vi "SensorsOperations.vi"(8 "ErrorIn":errorcluster, 9 "Operation":T1, 10 "RawAccelerationData In":dbl[][](array[numeric]), 11 "frame length ms":i64=50) -> (0 "ErrorOut":errorcluster, 1 "Tachometer Data":dbl[](array[numeric]), 2 "Normalized Acceleration Data":dbl[][](array[numeric]), 3 "RawAccelerationData Out":dbl[][](array[numeric]))   [LabVIEW 2019]
uses:
  Operation.ctl
  <vilib>/myRIO/Instrument Drivers/Onboard IO/AI/typedefs/AI Reference.ctl
  <vilib>/myRIO/Common/Instrument Driver Framework/Utilities/typedefs/myRIO Generic Hardware Reference.ctl
  <vilib>/myRIO/Common/Instrument Driver Framework/Utilities/typedefs/Hardware Version Enum.ctl
  <vilib>/myRIO/Common/Instrument Driver Framework/Utilities/typedefs/myRIO v1.0 Reference.ctl
  <vilib>/myRIO/Common/Instrument Driver Framework/Utilities/typedefs/Generic FPGA Reference.ctl
  <vilib>/myRIO/Common/Instrument Driver Framework/myRIO v1.0/AI/typedefs/AI Channels List.ctl
  <vilib>/myRIO/Common/Instrument Driver Framework/myRIO v1.0/AI/typedefs/AI Channels Enum.ctl
  <vilib>/myRIO/Common/Instrument Driver Framework/Utilities/typedefs/Analog Scaling Constants List.ctl
  <vilib>/myRIO/Common/Instrument Driver Framework/Utilities/typedefs/Analog Scaling Constants.ctl
  <vilib>/userdefined/High Color/nirio_resource_hc.ctl
  <vilib>/Platform/TimedLoop/XDataNode/timing_clust.ctl
  <vilib>/Platform/TimedLoop/XDataNode/nitl_modes.ctl
  <vilib>/Platform/TimedLoop/XDataNode/wakeup.ctl
  <vilib>/myRIO/Instrument Drivers/Onboard IO/I2C/typedefs/I2C Reference.ctl
  <vilib>/myRIO/Common/Instrument Driver Framework/myRIO v1.0/I2C/typedefs/I2C Channels Enum.ctl
  <vilib>/myRIO/Instrument Drivers/Onboard IO/I2C/typedefs/I2C Configuration.ctl
  <vilib>/myRIO/Instrument Drivers/Onboard IO/I2C/typedefs/I2C Transfer Rate.ctl
  <vilib>/myRIO/Common/Instrument Driver Framework/myRIO v1.0/AI/vis/myRIO v1.1 Open Throughput AI.vi
  <vilib>/myRIO/Common/Instrument Driver Framework/Utilities/vis/Validate Channels.vi
  <vilib>/myRIO/Common/Instrument Driver Framework/myRIO v1.0/AI/vis/myRIO v1.0 Reserve AI.vi
  <vilib>/myRIO/Common/Instrument Driver Framework/myRIO v1.0/I2C/vis/myRIO v1.0 Close I2C.vi
  <vilib>/myRIO/Common/Instrument Driver Framework/myRIO v1.0/AI/vis/myRIO v1.0 Close AI.vi
  <vilib>/myRIO/Common/Instrument Driver Framework/myRIO v1.0/AI/vis/myRIO v1.0 Build MUX Configuration AI.vi
  <vilib>/myRIO/Common/Instrument Driver Framework/myRIO v1.0/Resource Manager/vis/myRIO v1.0 Reserve Channel List.vi
  <vilib>/myRIO/Common/Instrument Driver Framework/myRIO v1.0/I2C/vis/myRIO v1.0 Unreserve I2C.vi
  <vilib>/myRIO/Common/Instrument Driver Framework/myRIO v1.0/AI/vis/myRIO v1.0 Unreserve AI.vi
  <vilib>/myRIO/Common/Instrument Driver Framework/myRIO v1.0/Resource Manager/vis/myRIO v1.0 Reserve Channel.vi
  <vilib>/myRIO/Common/Instrument Driver Framework/myRIO v1.0/Resource Manager/vis/myRIO v1.0 Unreserve Channel.vi
  <vilib>/myRIO/Common/Instrument Driver Framework/myRIO v1.0/I2C/vis/myRIO v1.0 Build MUX Configuration I2C.vi
  <vilib>/myRIO/Common/Instrument Driver Framework/myRIO v1.0/Resource Manager/vis/myRIO v1.0 Unreserve Channel List.vi
  <vilib>/myRIO/Common/Instrument Driver Framework/myRIO v1.0/Resource Manager/vis/myRIO v1.0 Build Mutex Name.vi
  <vilib>/myRIO/Common/Instrument Driver Framework/myRIO v1.0/Resource Manager/vis/myRIO v1.0 Create Configuration List.vi
  <vilib>/Utility/VariantDataType/GetNumericInfo.vi
  <vilib>/Utility/error.llb/Error Cluster From Error Code.vi
  <vilib>/myRIO/Common/Instrument Driver Framework/myRIO v1.0/myRIO v1.1 Open Throughput.vi
  <vilib>/myRIO/Common/Instrument Driver Framework/myRIO v1.0/AI/vis/myRIO v1.0 Get Scaling Constants AI.vi
  <vilib>/myRIO/Common/Instrument Driver Framework/Utilities/vis/IO Manager.vi
  <vilib>/myRIO/Common/Instrument Driver Framework/Utilities/vis/Configuration Manager.vi
  <vilib>/myRIO/Common/Instrument Driver Framework/myRIO v1.0/myRIO v1.0 Close.vi
  <vilib>/myRIO/Common/Instrument Driver Framework/myRIO v1.0/AI/vis/myRIO v1.0 Read AI.vi
  <vilib>/myRIO/Common/Instrument Driver Framework/myRIO v1.0/I2C/vis/myRIO v1.0 Shutdown I2C.vi
  <vilib>/myRIO/Common/Instrument Driver Framework/myRIO v1.0/Resource Manager/vis/myRIO v1.0 Configure IO.vi
  <vilib>/myRIO/Instrument Drivers/Onboard IO/AI/vis/myRIO AI Open.xnode
  <vilib>/platform/TimedLoop/XDataNode/XDataNode.xnode
  <vilib>/myRIO/Instrument Drivers/Onboard IO/I2C/typedefs/I2C User Configuration.ctl
  <vilib>/myRIO/Instrument Drivers/Onboard IO/I2C/I2C.lvlib
  <vilib>/myRIO/Instrument Drivers/Onboard IO/I2C/vis/myRIO I2C Open.xnode
  <vilib>/myRIO/Instrument Drivers/Onboard IO/AI/AI.lvlib
  <vilib>/Platform/TimedLoop/XDataNode/XDNodeRunTimeDep.lvlib
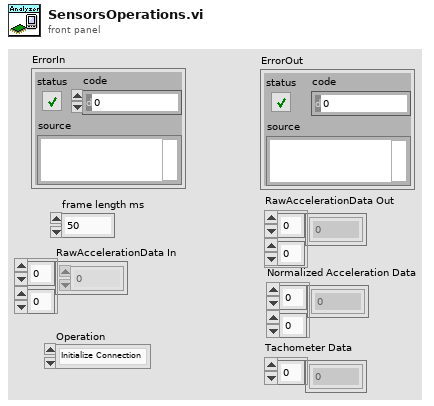
[diagram p1: front panel]
types:
  T1 = typedef "Operation.ctl" = enum16{"Initialize Connection", "Read Data", "Close Connection", "Calculate Data To g"}
  T2 = typedef "AnalyzerSettings.ctl" = cluster{"Create NS Timeout Code":i32, "Destroy NS Timeout Code":i32, "All threads":T3[], "AnalysisSettings":T4}
  T3 = typedef "AThreads.ctl" = enum16{"UI", "analyzeAccelerationData", "aquireAccelerationData", "communicateWebServices", "TDMSmanager", "aquireTachoSignal"}
  T4 = typedef "AnalysisSettings.ctl" = cluster{"Fault Thresholds":T5, "Analysis series name":string, "Save data analysis?":bool, "Band size":i32, "OrderAnalysis?":bool, "Accelerometer":T7, "fs [Hz]":dbl}
  T5 = typedef "Thresholds.ctl" = cluster{"Parameters labels":T6[], "Parameters thresholds":dbl[], "Freqs and thresholds":dbl[][], "Orders and thresholds":dbl[][]}
  T6 = typedef "FaultParameter.ctl" = enum16{"Kurtosis", "RMS", "Crest factor"}
  T7 = typedef "Accelerometer.ctl" = enum16{"None", "MPU6050", "MMA7351"}
  T8 = typedef "nirio_resource_hc.ctl" = tag
  T9 = typedef "Hardware Version Enum.ctl" = enum16{"Unknown", "myRIO-1900", "myRIO-1950", "roboRIO", "NI ELVIS RIO CM", "ELVIS III"}
  T10 = typedef "XDNodeRunTimeDep.lvlib/timing_clust.ctl" = cluster{"Expected End [f-1]":u64, "Actual End [f-1]":u64, "Finished Late? [f-1]":bool, "Expected End [i-1]":u64, "Actual End [i-1]":u64, "Finished Late? [i-1]":bool, "Expected Start [i]":u64, "Actual Start [i]":u64, "Expected Start [f]":u64, "Actual Start [f]":u64, "Source Name":string, "Structure Name":string, "Period":i64, "Deadline":i64, "Offset":i64, "Start":i64, "Priority":i32, "Timeout":i32, "Mode":T11, "Wakeup Reason":T12, "Error":errorcluster, "Source Type":string, "Secondary Source Type":string, "Global End Time":u64, "Global Start Time":u64, "Frame Duration":u64, "Iteration Duration":u64, "Assigned CPU":i32, "I/O Scan Engine Mode":u32}
  T11 = typedef "XDNodeRunTimeDep.lvlib/nitl_modes.ctl" = enum32{"No Change", "Process missed periods, maintain original phase", "Discard missed periods, maintain original phase", "Process missed periods, ignore original phase", "Discard missed periods, ignore original phase"}
  T12 = typedef "XDNodeRunTimeDep.lvlib/wakeup.ctl" = enum32{"Normal", "Aborted", "Asynchronous wakeup", "Timing source error", "Timed loop error", "Timeout"}
  T13 = typedef "I2C.lvlib/I2C Reference.ctl" = cluster{"myRIO Reference":T14, "I2C Channels Enum":T17, "I2C Configuration":T18}
  T14 = typedef "myRIO Generic Hardware Reference.ctl" = cluster{"myRIO Model":T9, "myRIO Hardware Reference":T15}
  T15 = typedef "myRIO v1.0 Reference.ctl" = cluster{"Generic FPGA Reference":T16, "Allow multiple opens":bool}
  T16 = typedef "Generic FPGA Reference.ctl" = refnum<k20>
  T17 = typedef "I2C Channels Enum.ctl" = enum16{"Not Connected", "A/I2C", "B/I2C", "I2C/I2C"}
  T18 = typedef "I2C.lvlib/I2C Configuration.ctl" = cluster{"I2C Transfer Rate":T19}
  T19 = typedef "I2C.lvlib/I2C Transfer Rate.ctl" = enum16{"Standard mode (100 kbps)", "Fast mode (400 kbps)"}
  T20 = typedef "AI.lvlib/AI Reference.ctl" = cluster{"myRIO Reference":T14, "AI Channels List":T21, "AI Scaling Constants List":T23}
  T21 = typedef "AI Channels List.ctl" = T22[]
  T22 = typedef "AI Channels Enum.ctl" = enum16{"Not Connected", "AudioIn/Left", "AudioIn/Right", "C/AI0", "C/AI1", "A/AI0", "A/AI1", "A/AI2", "A/AI3", "A/AI4", "A/AI5", "A/AI6", "A/AI7", "B/AI0", "B/AI1", "B/AI2", "B/AI3", "B/AI4", "B/AI5", "B/AI6", "B/AI7", "AI/AI0", "AI/AI1", "AI/AI2", "AI/AI3", "A/AI0 (DIFF)", "A/AI1 (DIFF)", "A/AI2 (DIFF)", "A/AI3 (DIFF)", "B/AI0 (DIFF)", "B/AI1 (DIFF)", "B/AI2 (DIFF)", "B/AI3 (DIFF)"}
  T23 = typedef "Analog Scaling Constants List.ctl" = T24[]
  T24 = typedef "Analog Scaling Constants.ctl" = cluster{"LSB Weight (Volts)":dbl, "Offset (Volts)":dbl, "Signed?":bool}
  T25 = typedef "I2C.lvlib/I2C User Configuration.ctl" = cluster{"I2C Transfer Rate":T19}
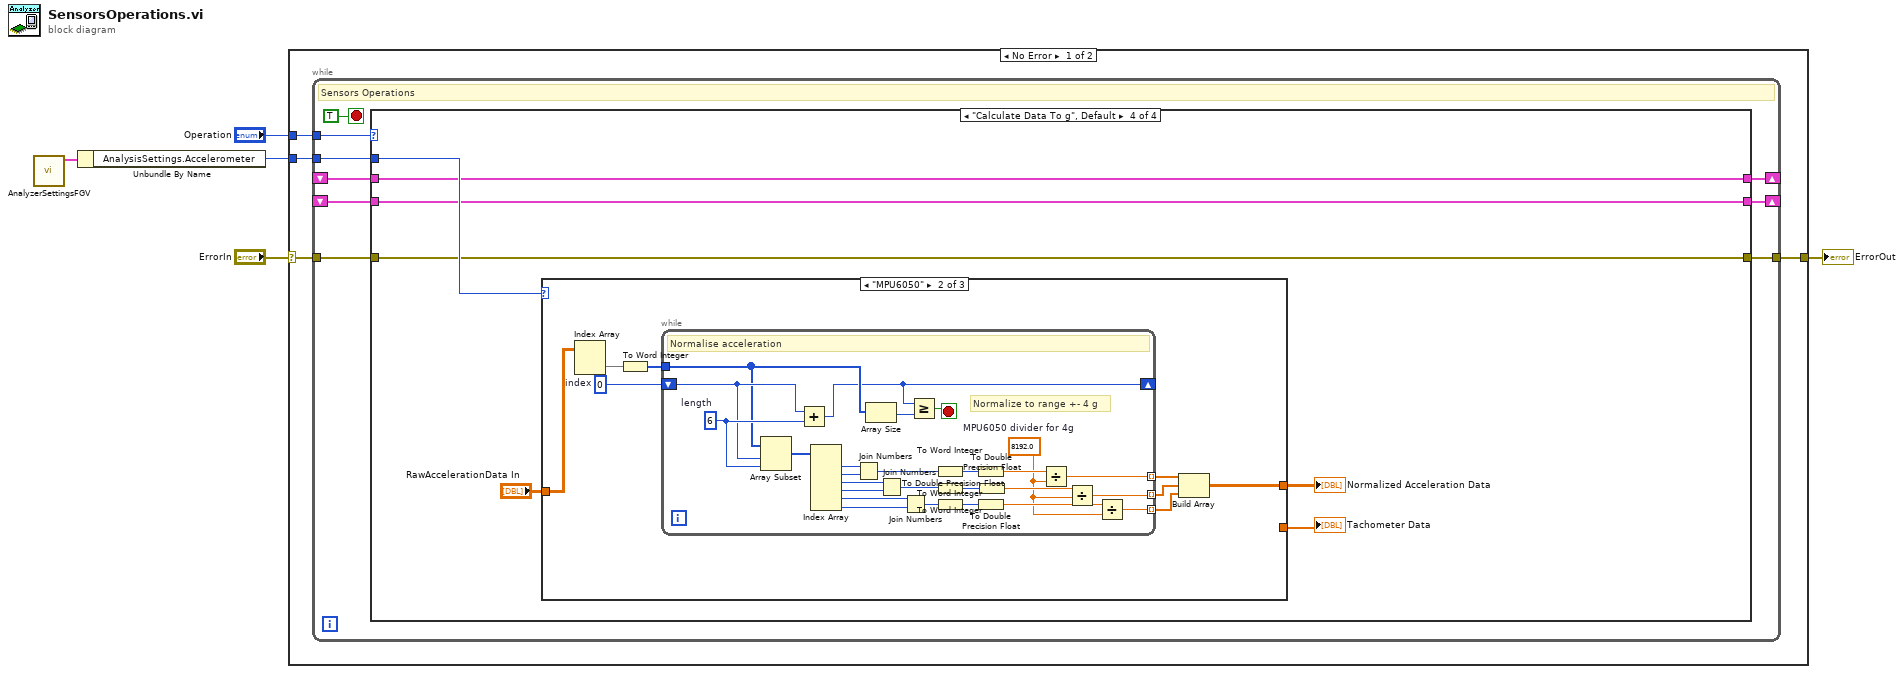
[diagram p0: block diagram]
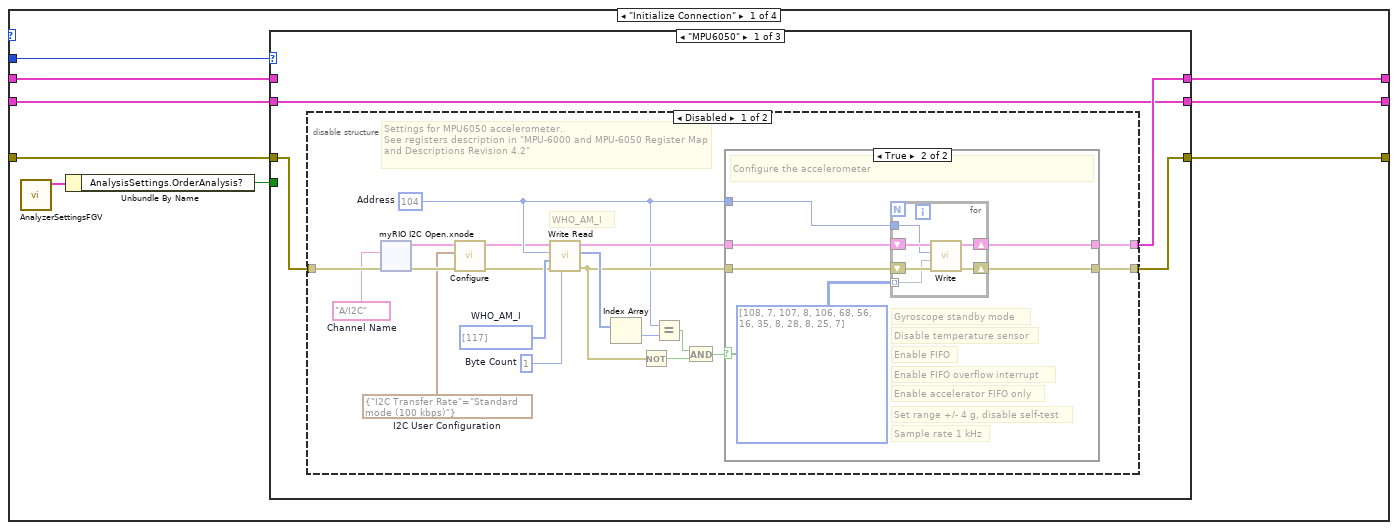
[diagram p2: hidden frame]
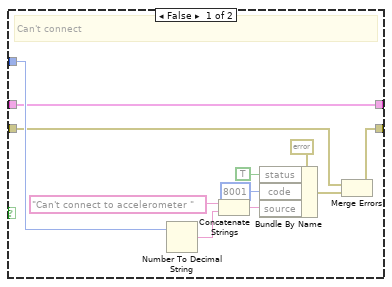
[diagram p3: hidden frame]
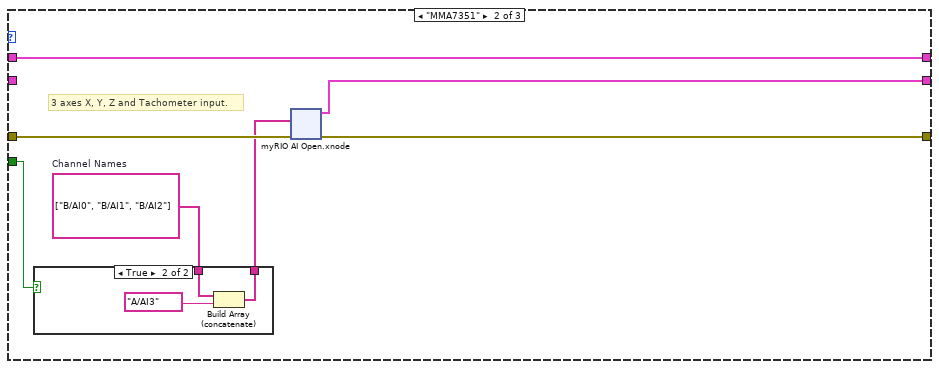
[diagram p5: hidden frame]
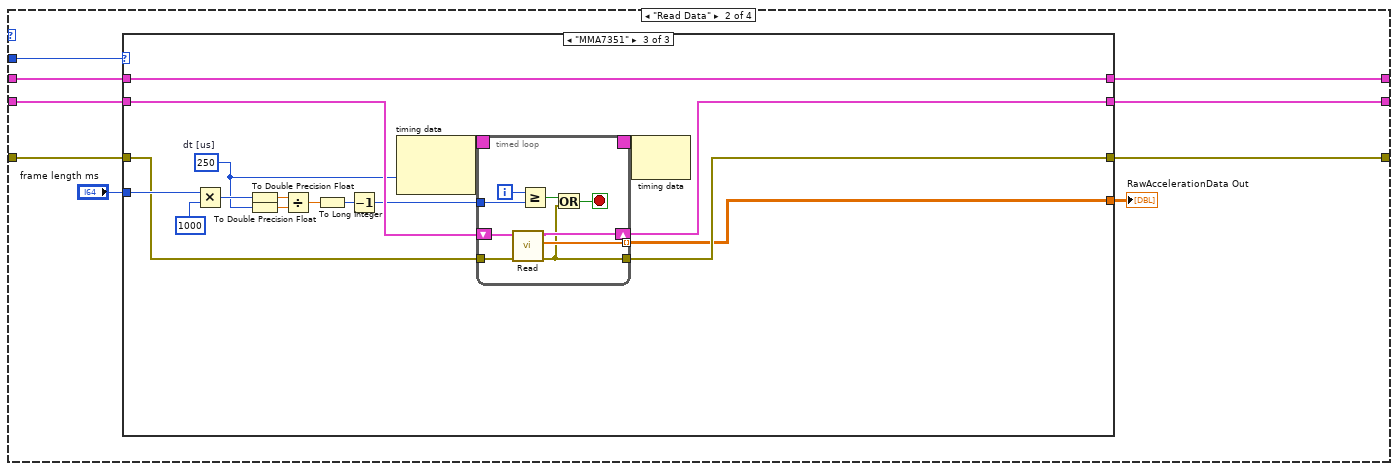
[diagram p8: hidden frame]
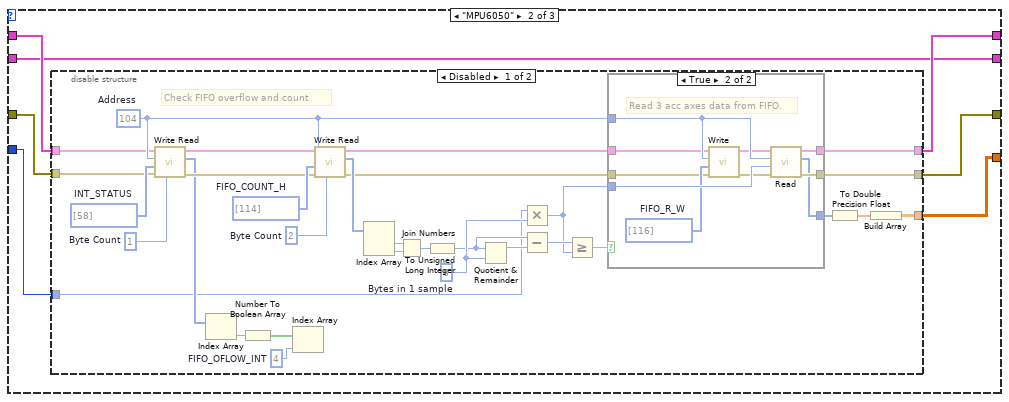
[diagram p10: hidden frame]
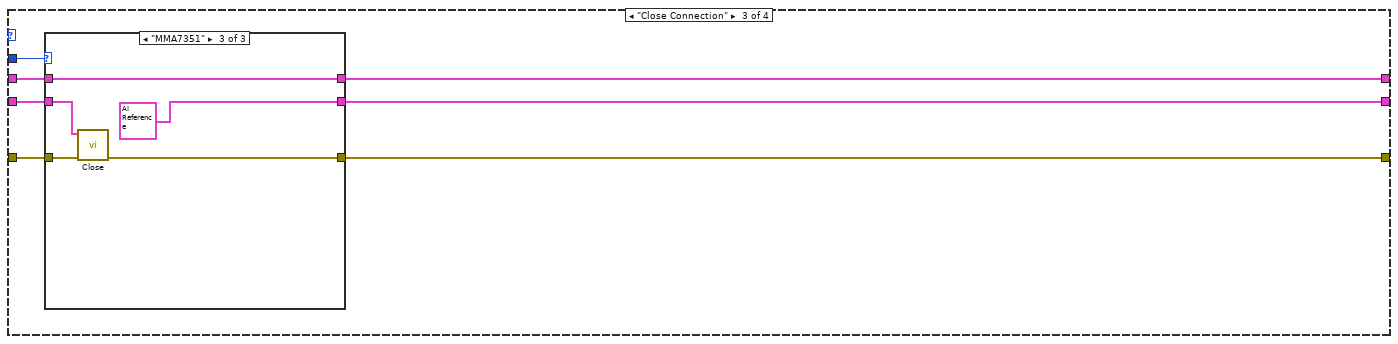
[diagram p13: hidden frame]
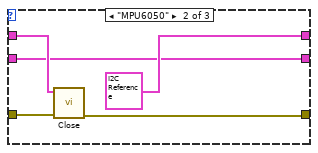
[diagram p15: hidden frame]
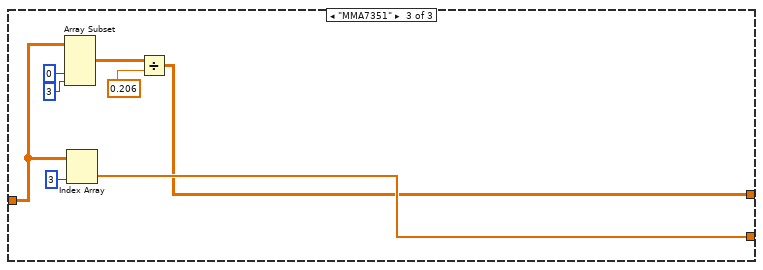
[diagram p17: hidden frame]
diagram:
  n1 = call "AnalyzerSettingsFGV.vi"() -> ("GlobalSettingsOut"=w3:T2)  [unwired: 11 in]
  n2 = Unbundle By Name(w3) -> ("AnalysisSettings.Accelerometer"=w2:T7)
  n3 = case shown="No Error" "ErrorIn" {
    selector: "ErrorIn" -> [w6 w272]
    tunnel: "Operation" -> [w9 _]
    tunnel: [w8 w272] -> w4
    tunnel: w2 -> [w7 _]
    frame No Error {
      n4 = while {
        tunnel: w9 -> [w17]
        tunnel: w7 -> [w16]
        shift-right: [w12] -> _
        shift-left: _ -> [w13]
        shift-right: [w11] -> _
        shift-left: _ -> [w10]
        tunnel: w6 -> [w15]
        tunnel: [w14] -> w8
        stop <- TRUE stop-if-true
        # "Sensors Operations"
        n5 = case shown="\"Calculate Data To g\", Default" w17 {
          tunnel: w16 -> [w27 w115 w208 w228]
          tunnel: w15 -> [w26 w113 w204 w224]
          tunnel: [w25 w114 w205 w224] -> w14
          tunnel: w13 -> [w24 w112 w207 w222]
          tunnel: [w23 w109 w202 w222] -> w12
          tunnel: [w22 w108 w203 w223] -> w11
          tunnel: w10 -> [w21 w111 w206 w223]
          frame "Initialize Connection" {
            n6 = call "AnalyzerSettingsFGV.vi"() -> ("GlobalSettingsOut"=w20:T2)  [unwired: 11 in]
            n7 = Unbundle By Name(w20) -> ("AnalysisSettings.OrderAnalysis?"=w19:bool)
            n8 = case shown="\"MPU6050\"" w27 {
              tunnel: w26 -> [w30 w81 w106]
              tunnel: [w29 w80 w106] -> w25
              tunnel: w24 -> [_ w75 w104]
              tunnel: [w31 w75 w104] -> w23
              tunnel: [w28 w79 w105] -> w22
              tunnel: w21 -> [w28 _ w105]
              tunnel: w19 -> [_ w78 _]
              frame "MPU6050" {
                n9 = disable-structure shown="Disabled" {
                  disable-tunnel: [w40 _] -> w31
                  disable-tunnel: w30 -> [w39 w74]
                  disable-tunnel: [w32 w74] -> w29
                  frame Disabled {
                    w33 = T25 {"I2C Transfer Rate"=enum."Standard mode (100 kbps)"}  # I2C User Configuration
                    w38 = tag "A/I2C"  # Channel Name
                    w42 = u8 104  # Address
                    w48 = u32 1  # Byte Count
                    w47 = u8[] [117]  # WHO_AM_I
                    # "Settings for MPU6050 accelerometer.\nSee registers description in \"MPU-6000 and MPU-6050 Register Map and Descriptions Revision 4.2\""
                    # "WHO_AM_I"
                    n10 = xnode "myRIO I2C Open.xnode"("error in (no error)"=w39, "Channel Name"=w38) -> ("error out"=w36:errorcluster, "I2C Ref Out"=w37:T13)  [unwired: 1 in]
                    n11 = call <vilib>:"Configure.vi"("error in (no error)"=w36, "I2C User Configuration"=w33, "I2C Ref In"=w37) -> ("error out"=w34:errorcluster, "I2C Ref Out"=w35:T13)  [unwired: 7 in]
                    n12 = call <vilib>:"Write Read.vi"("Byte Count"=w48, "error in (no error)"=w34, "Bytes to Write"=w47, "Slave Address (7-bit)"=w42, "I2C Ref In"=w35) -> ("error out"=w44:errorcluster, "Bytes Read"=w49:u8[], "I2C Ref Out"=w46:T13)  [unwired: 3 in]
                    n13 = Index Array(array=w49) -> (element=w50:u8)  [unwired: 1 in]
                    n14 = Not(x=w44) -> (.not. x?=w43:bool)
                    n15 = Equal?(x=w42, y=w50) -> (x = y?=w45:bool)
                    n16 = And(x=w45, y=w43) -> (x .and. y?=w41:bool)
                    n17 = case shown="True" w41 {
                      tunnel: w42 -> [w59 w64]
                      tunnel: w46 -> [w52 w67]
                      tunnel: w44 -> [w54 w66]
                      tunnel: [w51 w63] -> w32
                      tunnel: [w52 w62] -> w40
                      frame False {
                        # "Can't connect"
                        n18 = Number To Decimal String(number=w59) -> (decimal integer string=w56:string)  [unwired: 1 in]
                        n19 = Concatenate Strings("Can't connect to accelerometer " ("source"), w56) -> (w58:string)
                        n20 = Bundle By Name(cluster=errorcluster {"status"=FALSE, "code"=0, "source"=""} ("error constant"), "status"=TRUE, "code"=8001, "source"=w58) -> (w53:errorcluster)
                        n21 = Merge Errors(w54, w53) -> (w51:errorcluster)
                      }
                      frame True {
                        # "Sample rate 1 kHz"
                        # "Enable accelerator FIFO only"
                        # "Disable temperature sensor"
                        # "Gyroscope standby mode"
                        # "Set range +/- 4 g, disable self-test"
                        # "Enable FIFO"
                        # "Enable FIFO overflow interrupt"
                        # "Configure the accelerometer"
                        n22 = for {
                          shift-right: [w70] -> w63
                          shift-left: w66 -> [w73]
                          shift-right: [w71] -> w62
                          shift-left: w67 -> [w72]
                          tunnel: u8[][] [[108, 7], [107, 8], [106, 68], [56, 16], [35, 8], [28, 8], [25, 7]] ("Bytes to Write") -> [w69] mode=indexing
                          tunnel: w64 -> [w68]
                          n23 = call <vilib>:"Write.vi"("error in (no error)"=w73, "Bytes to Write"=w69, "Slave Address (7-bit)"=w68, "I2C Ref In"=w72) -> ("error out"=w70:errorcluster, "I2C Ref Out"=w71:T13)  [unwired: 6 in]
                        }
                      }
                    }
                  }
                  frame Enabled {
                  }
                }
              }
              frame "MMA7351" {
                w77 = tag[] ["B/AI0", "B/AI1", "B/AI2"]  # Channel Names
                # "3 axes X, Y, Z and Tachometer input."
                n24 = case shown="True" w78 {
                  tunnel: w77 -> [w82 w85]
                  tunnel: [w82 w83] -> w76
                  frame False {
                  }
                  frame True {
                    n25 = Build Array (concatenate)(w85, tag "A/AI3" ("myRIO AI Channel")) -> (w83:tag[])
                  }
                }
                n26 = xnode "myRIO AI Open.xnode"("error in (no error)"=w81, "Channel Names"=w76) -> ("error out"=w80:errorcluster, "AI Ref Out"=w79:T20)  [unwired: 1 in]
              }
              frame "None", Default {
              }
            }
          }
          frame "Read Data" {
            n27 = case shown="\"MMA7351\"" w115 {
              tunnel: [w118 w119 w173] -> w114
              tunnel: w113 -> [w118 w121 w175]
              tunnel: w112 -> [w116 w124 w170]
              tunnel: w111 -> [w117 w120 w177]
              tunnel: "frame length ms" -> [_ w125 w180]
              tunnel: [w116 w123 w170] -> w109
              tunnel: [_ w122 w172] -> w107
              tunnel: [w117 w120 w174] -> w108
              frame "None", Default {
              }
              frame "MPU6050" {
                n28 = disable-structure shown="Disabled" {
                  disable-tunnel: w121 -> [w133 w168]
                  disable-tunnel: w125 -> [w132 _]
                  disable-tunnel: [w131 w168] -> w119
                  disable-tunnel: w124 -> [w130 w169]
                  disable-tunnel: [w129 w169] -> w123
                  disable-tunnel: [w126 _] -> w122
                  frame Disabled {
                    w145 = 4  # FIFO_OFLOW_INT
                    w148 = u32 1  # Byte Count
                    w149 = u8[] [58]  # INT_STATUS
                    w139 = u32 6  # Bytes in 1 sample
                    w154 = u8[] [114]  # FIFO_COUNT_H
                    w140 = u8 104  # Address
                    w155 = u32 2  # Byte Count
                    # "Check FIFO overflow and count"
                    n29 = call <vilib>:"Write Read.vi"("Byte Count"=w148, "error in (no error)"=w133, "Bytes to Write"=w149, "Slave Address (7-bit)"=w140, "I2C Ref In"=w130) -> ("error out"=w150:errorcluster, "Bytes Read"=w144:u8[], "I2C Ref Out"=w151:T13)  [unwired: 3 in]
                    n30 = Index Array(array=w144) -> (element=w147:u8)  [unwired: 1 in]
                    n31 = Number To Boolean Array(number=w147) -> (Boolean array=w146:bool[])
                    n32 = Index Array(array=w146, index=w145) -> ()  [unwired: 1 out]
                    n33 = call <vilib>:"Write Read.vi"("Byte Count"=w155, "error in (no error)"=w150, "Bytes to Write"=w154, "Slave Address (7-bit)"=w140, "I2C Ref In"=w151) -> ("error out"=w136:errorcluster, "Bytes Read"=w153:u8[])  [unwired: 3 in, 1 out]
                    n34 = Index Array(array=w153) -> (element #1=w152:u8, element #2=w141:u8)  [unwired: 2 in]
                    n35 = Join Numbers(hi=w152, lo=w141) -> ((hi.lo)=w142:u16)
                    n36 = To Unsigned Long Integer(number=w142) -> (unsigned 32bit integer=w135:u32)
                    n37 = Quotient & Remainder(x=w135, y=w139) -> (x-y*floor(x/y)=w143:u32)  [unwired: 1 out]
                    n38 = Multiply(x=w132, y=w139) -> (x*y=w137:i64)
                    n39 = Subtract(x=w135, y=w143) -> (x-y=w138:u32)
                    n40 = Greater Or Equal?(x=w138, y=w137) -> (x >= y?=w134:bool)
                    n41 = case shown="True" w134 {
                      tunnel: [w157 w160] -> w131
                      tunnel: w140 -> [_ w164]
                      tunnel: w136 -> [w157 w165]
                      tunnel: w137 -> [_ w167]
                      tunnel: w130 -> [w156 w163]
                      tunnel: [w156 w159] -> w129
                      tunnel: [_ w158] -> w128
                      frame False {
                      }
                      frame True {
                        w166 = u8[] [116]  # FIFO_R_W
                        # "Read 3 acc axes data from FIFO."
                        n42 = call <vilib>:"Write.vi"("error in (no error)"=w165, "Bytes to Write"=w166, "Slave Address (7-bit)"=w164, "I2C Ref In"=w163) -> ("error out"=w162:errorcluster, "I2C Ref Out"=w161:T13)  [unwired: 6 in]
                        n43 = call <vilib>:"Read.vi"("error in (no error)"=w162, "Byte Count"=w167, "Slave Address (7-bit)"=w164, "I2C Ref In"=w161) -> ("error out"=w160:errorcluster, "Bytes Read"=w158:u8[], "I2C Ref Out"=w159:T13)  [unwired: 4 in]
                      }
                    }
                    n44 = To Double Precision Float(number=w128) -> (double precision float=w127:dbl[])
                    n45 = Build Array(w127) -> (w126:dbl[][])
                  }
                  frame Enabled {
                  }
                }
              }
              frame "MMA7351" {
                w171 = i64 250  # dt [us]
                n46 = Multiply(x=w180, y=i64 1000) -> (x*y=w182:i64)
                n47 = To Double Precision Float(number=w182) -> (double precision float=w183:dbl)
                n48 = To Double Precision Float(number=w171) -> (double precision float=w184:dbl)
                n49 = Divide(x=w183, y=w184) -> (x/y=w185:dbl)
                n50 = To Long Integer(number=w185) -> (32bit integer=w186:i32)
                n51 = Decrement(x=w186) -> (x-1=w176:i32)
                n52 = node-c288(w171) -> (w179:T10)  [unwired: 1 in]
                n53 = timed-loop {
                  timing: w179 -> [_]
                  timing-out: [_] -> w178
                  tunnel: w175 -> [w192]
                  tunnel: [w187] -> w173
                  tunnel: [w190] -> w172 mode=indexing
                  tunnel: w176 -> [w189]
                  shift-right: [w191] -> w174
                  shift-left: w177 -> [w193]
                  i -> [w194]
                  stop <- w188 stop-if-true
                  n54 = call <vilib>:"Read.vi"("error in (no error)"=w192, "AI Ref In"=w193) -> ("error out"=w187:errorcluster, "Values"=w190:dbl[], "AI Ref Out"=w191:T20)  [unwired: 7 in]
                  n55 = Greater Or Equal?(x=w194, y=w189) -> (x >= y?=w195:bool)
                  n56 = Or(x=w195, y=w187) -> (x .or. y?=w188:bool)
                }
                n57 = node-c288(w178) -> ()  [unwired: 1 out]
              }
            }
            "RawAccelerationData Out" <- w107
          }
          frame "Close Connection" {
            n58 = case shown="\"MMA7351\"" w208 {
              tunnel: w207 -> [w209 w215 w217]
              tunnel: w206 -> [w210 w212 w220]
              tunnel: [w211 w214 w219] -> w205
              tunnel: w204 -> [w211 w216 w221]
              tunnel: [w210 w212 T20 {"myRIO Reference"={"myRIO Model"=enum."Unknown", "myRIO Hardware Reference"={"Generic FPGA Reference"=refnum, "Allow multiple opens"=FALSE}}, "AI Channels List"=[], "AI Scaling Constants List"=[]} ("AI Ref Out")] -> w203
              tunnel: [w209 T13 {"myRIO Reference"={"myRIO Model"=enum."Unknown", "myRIO Hardware Reference"={"Generic FPGA Reference"=refnum, "Allow multiple opens"=FALSE}}, "I2C Channels Enum"=enum."Not Connected", "I2C Configuration"={"I2C Transfer Rate"=enum."Standard mode (100 kbps)"}} ("I2C Ref Out") w217] -> w202
              frame "None", Default {
              }
              frame "MPU6050" {
                n59 = call <vilib>:"Close.vi"("error in (no error)"=w216, "I2C Ref In"=w215) -> ("error out"=w214:errorcluster)  [unwired: 9 in]
              }
              frame "MMA7351" {
                n60 = call <vilib>:"Close.vi"("error in (no error)"=w221, "AI Ref In"=w220) -> ("error out"=w219:errorcluster)  [unwired: 9 in]
              }
            }
          }
          frame "Calculate Data To g", Default {
            n61 = case shown="\"MPU6050\"" w228 {
              tunnel: "RawAccelerationData In" -> [w229 w234 w269]
              tunnel: [_ _ w270] -> w226
              tunnel: [w229 w230 w264] -> w225
              frame "None", Default {
              }
              frame "MPU6050" {
                w237 = 0  # index
                n62 = Index Array(array=w234) -> (element=w236:dbl[])  [unwired: 2 in]
                n63 = To Word Integer(number=w236) -> (16bit integer=w235:i16[])
                n64 = while {
                  tunnel: w235 -> [w244]
                  shift-right: [w241] -> _
                  shift-left: w237 -> [w262]
                  tunnel: [w240] -> w233 mode=indexing
                  tunnel: [w239] -> w231 mode=indexing
                  tunnel: [w238] -> w232 mode=indexing
                  stop <- w243 stop-if-true
                  w252 = 8192.0  # MPU6050 divider for 4g
                  w263 = 6  # length
                  # "Normalize to range +- 4 g"
                  # "Normalise acceleration"
                  n65 = Array Subset(array=w244, index=w262, length=w263) -> (w251:i16[])
                  n66 = Add(x=w262, y=w263) -> (x+y=w241:i32)
                  n67 = Index Array(array=w251) -> (element #1=w246:i16, element #2=w245:i16, element #3=w247:i16, element #4=w248:i16, element #5=w249:i16, element #6=w250:i16)  [unwired: 6 in]
                  n68 = Join Numbers(hi=w246, lo=w245) -> ((hi.lo)=w253:u32)
                  n69 = Array Size(array=w244) -> (size(s)=w242:i32)
                  n70 = Join Numbers(hi=w247, lo=w248) -> ((hi.lo)=w254:u32)
                  n71 = Join Numbers(hi=w249, lo=w250) -> ((hi.lo)=w255:u32)
                  n72 = Greater Or Equal?(x=w241, y=w242) -> (x >= y?=w243:bool)
                  n73 = To Word Integer(number=w253) -> (16bit integer=w256:i16)
                  n74 = To Word Integer(number=w254) -> (16bit integer=w257:i16)
                  n75 = To Word Integer(number=w255) -> (16bit integer=w258:i16)
                  n76 = To Double Precision Float(number=w256) -> (double precision float=w259:dbl)
                  n77 = To Double Precision Float(number=w258) -> (double precision float=w261:dbl)
                  n78 = To Double Precision Float(number=w257) -> (double precision float=w260:dbl)
                  n79 = Divide(x=w259, y=w252) -> (x/y=w240:dbl)
                  n80 = Divide(x=w260, y=w252) -> (x/y=w239:dbl)
                  n81 = Divide(x=w261, y=w252) -> (x/y=w238:dbl)
                }
                n82 = Build Array(w233, w231, w232) -> (w230:dbl[][])
              }
              frame "MMA7351" {
                n83 = Array Subset(array=w269, index (col)=0 ("index"), length (col)=3 ("length")) -> (w266:dbl[][])  [unwired: 2 in]
                n84 = Index Array(array=w269, index (col)=3 ("disabled index (col)")) -> (element=w270:dbl[])  [unwired: 1 in]
                n85 = Divide(x=w266, y=0.206) -> (x/y=w264:dbl[][])
              }
            }
            "Normalized Acceleration Data" <- w225
            "Tachometer Data" <- w226
          }
        }
      }
    }
    frame Error {
    }
  }
  "ErrorOut" <- w4
